vi "EXO_SignalRecord2.vi"(0 "V-1":bool, 1 "V-11":bool, 2 "V-12":bool, 3 "V-13":bool, 4 "V-6":bool, 5 "V-2":bool, 6 "V-7":bool, 7 "V-3":bool, 8 "V-8":bool, 9 "V-4":bool, 10 "V-9":bool, 11 "V-5":bool, 12 "V-14":bool, 14 "V-15":bool, 15 "V-10":bool) -> (13 "output cluster":T1)   [LabVIEW 2012]
panel:
  in  "stop":bool
  # "EXO DatabaseWrite Sub-VI (II)"
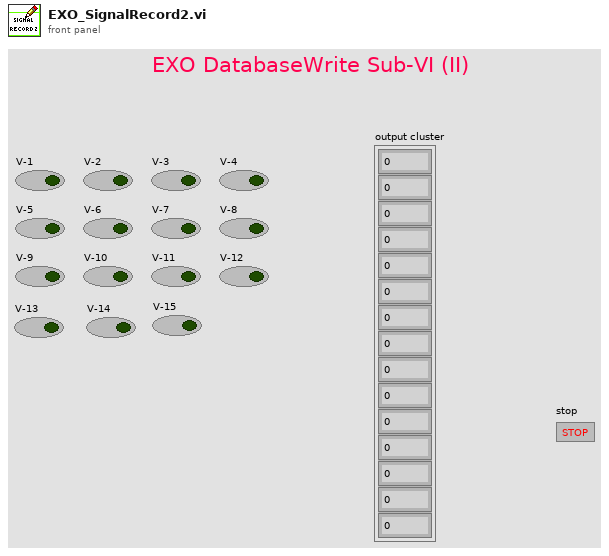
[diagram p1: front panel]
types:
  T1 = cluster{dbl, dbl, dbl, dbl, dbl, dbl, dbl, dbl, dbl, dbl, dbl, dbl, dbl, dbl, dbl}
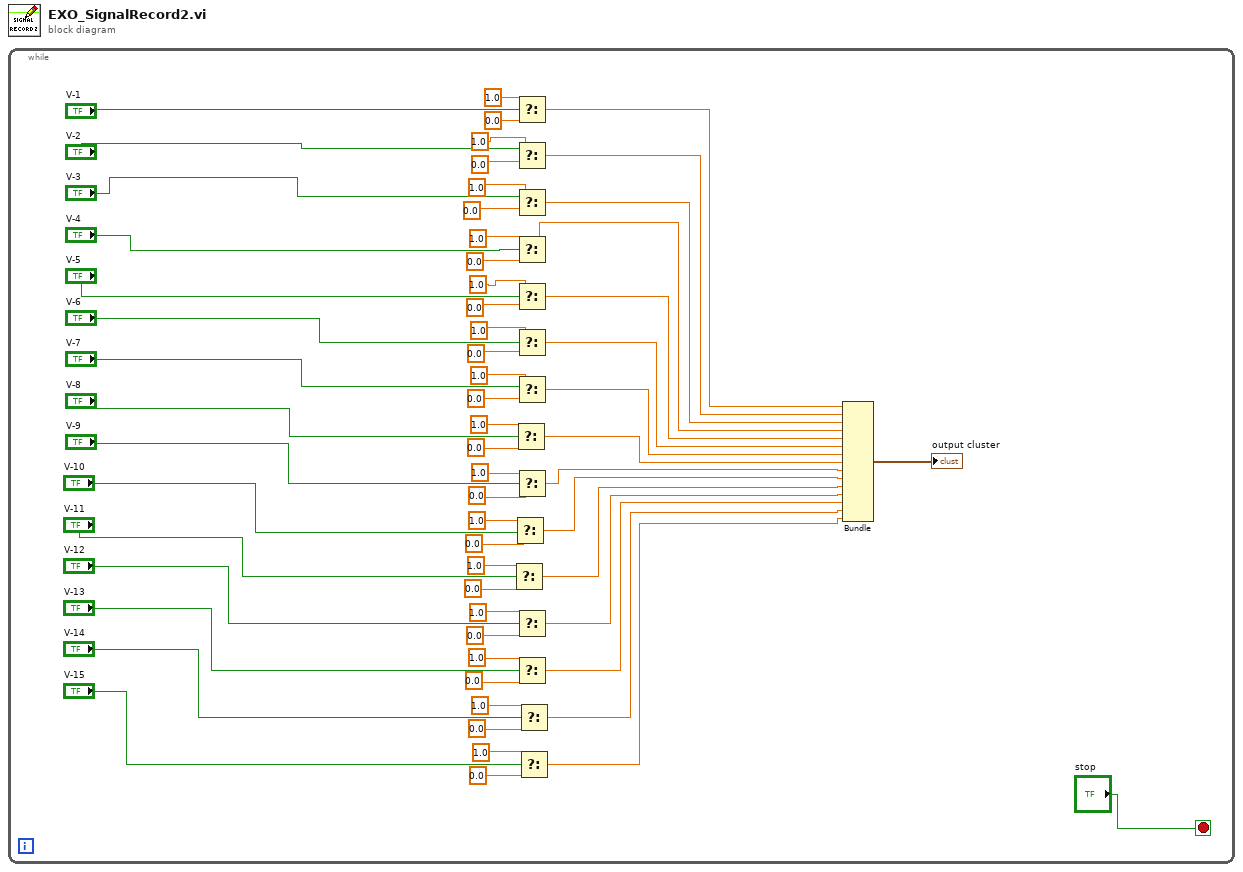
[diagram p0: block diagram]
diagram:
  n1 = while {
    stop <- "stop" stop-if-true
    n2 = Select(t=1.0, s="V-11", f=0.0) -> (s? t:f=w51:dbl)
    n3 = Select(t=1.0, s="V-10", f=0.0) -> (s? t:f=w52:dbl)
    n4 = Select(t=1.0, s="V-8", f=0.0) -> (s? t:f=w54:dbl)
    n5 = Select(t=1.0, s="V-1", f=0.0) -> (s? t:f=w61:dbl)
    n6 = Select(t=1.0, s="V-2", f=0.0) -> (s? t:f=w60:dbl)
    n7 = Select(t=1.0, s="V-3", f=0.0) -> (s? t:f=w59:dbl)
    n8 = Select(t=1.0, s="V-4", f=0.0) -> (s? t:f=w58:dbl)
    n9 = Select(t=1.0, s="V-5", f=0.0) -> (s? t:f=w57:dbl)
    n10 = Select(t=1.0, s="V-6", f=0.0) -> (s? t:f=w56:dbl)
    n11 = Select(t=1.0, s="V-7", f=0.0) -> (s? t:f=w55:dbl)
    n12 = Select(t=1.0, s="V-9", f=0.0) -> (s? t:f=w53:dbl)
    n13 = Select(t=1.0, s="V-12", f=0.0) -> (s? t:f=w50:dbl)
    n14 = Select(t=1.0, s="V-13", f=0.0) -> (s? t:f=w49:dbl)
    n15 = Select(t=1.0, s="V-14", f=0.0) -> (s? t:f=w48:dbl)
    n16 = Select(t=1.0, s="V-15", f=0.0) -> (s? t:f=w47:dbl)
    n17 = Bundle(w61, w60, w59, w58, w57, w56, w55, w54, w53, w52, w51, w50, w49, w48, w47) -> (→"output cluster":T1)  [unwired: 1 in]
  }
